vi "Planecontrolscrashworks.vi"() -> ()   [LabVIEW 2015]
uses:
  <vilib>/DAQmx/read.llb/DAQmx Read (Analog Wfm 1Chan NSamp).vi
  <vilib>/DAQmx/create/channels.llb/DAQmx Create Channel (AI-Voltage-Basic).vi
  <vilib>/DAQmx/configure/timing.llb/DAQmx Timing (Sample Clock).vi
  \\hs4.lboro.ac.uk\elhh3/LabVIEW Data/Work/Invictus/Global.vi
  <vilib>/DAQmx/miscellaneous.llb/DAQmx Fill In Error Info.vi
panel:
  in  "stop 4":bool
  out "Crash":bool
  in  "stop 5":bool
  in  "Amplitude":dbl(slide) scale=0.0..5000.0
  in  "stop 3":bool
  in  "stop 2":bool
  in  "stop":bool
  out "Altitude":dbl
  out "Iterations":i32
  out "Light Sensor":dbl
  out "Roll":dbl
  out "Airspeed":dbl
  out "Boolean":bool
  in  "Wing Tips":bool
  out "Previous Speed":dbl
  out "?":bool
  out "?":bool
  out "?":bool
  out "?":bool
  in  "Current Speed":dbl(slide) scale=0.0..400.0
  in  "Roll Slider":dbl(slide) scale=-90.0..90.0
  in  "Fan":bool
  in  "Breaks":bool
  in  "Right Indicator":bool
  in  "Left Indicator":bool
  out "Waveform Graph":waveform(dbl)(graph)
  in  "?":bool
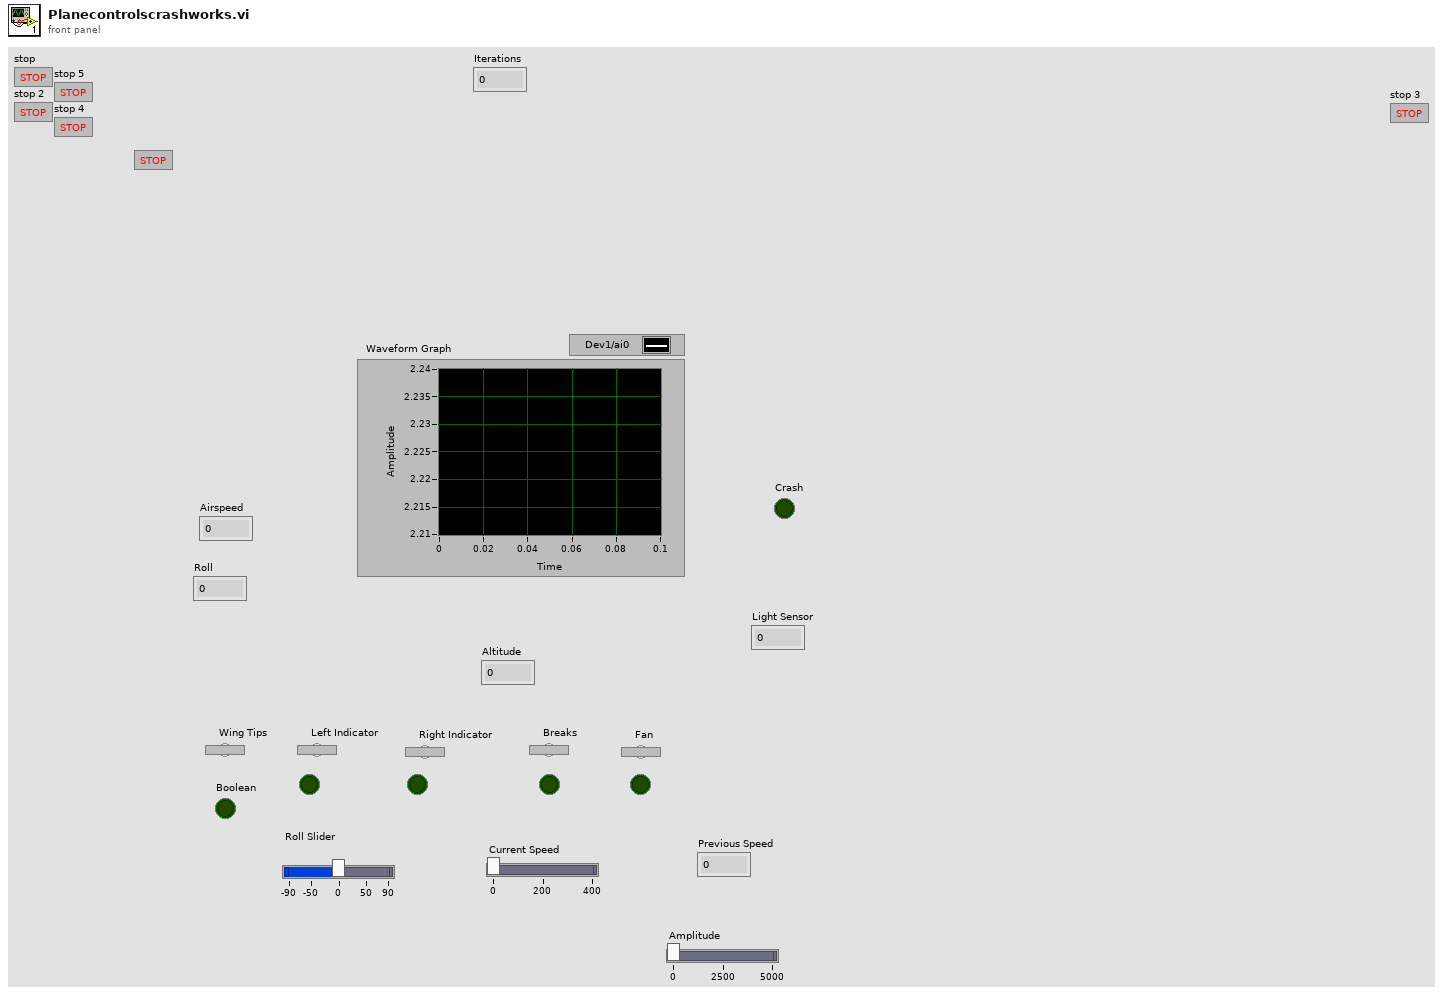
[diagram p1: front panel]
types:
  T1 = cluster{"Airspeed":dbl, "Altitude":dbl, "Vertical Speed":dbl, "Pitch":dbl, "Roll":dbl, "Heading":dbl, "Turn Indicator":dbl, "Latitude":dbl, "Longitude":dbl}
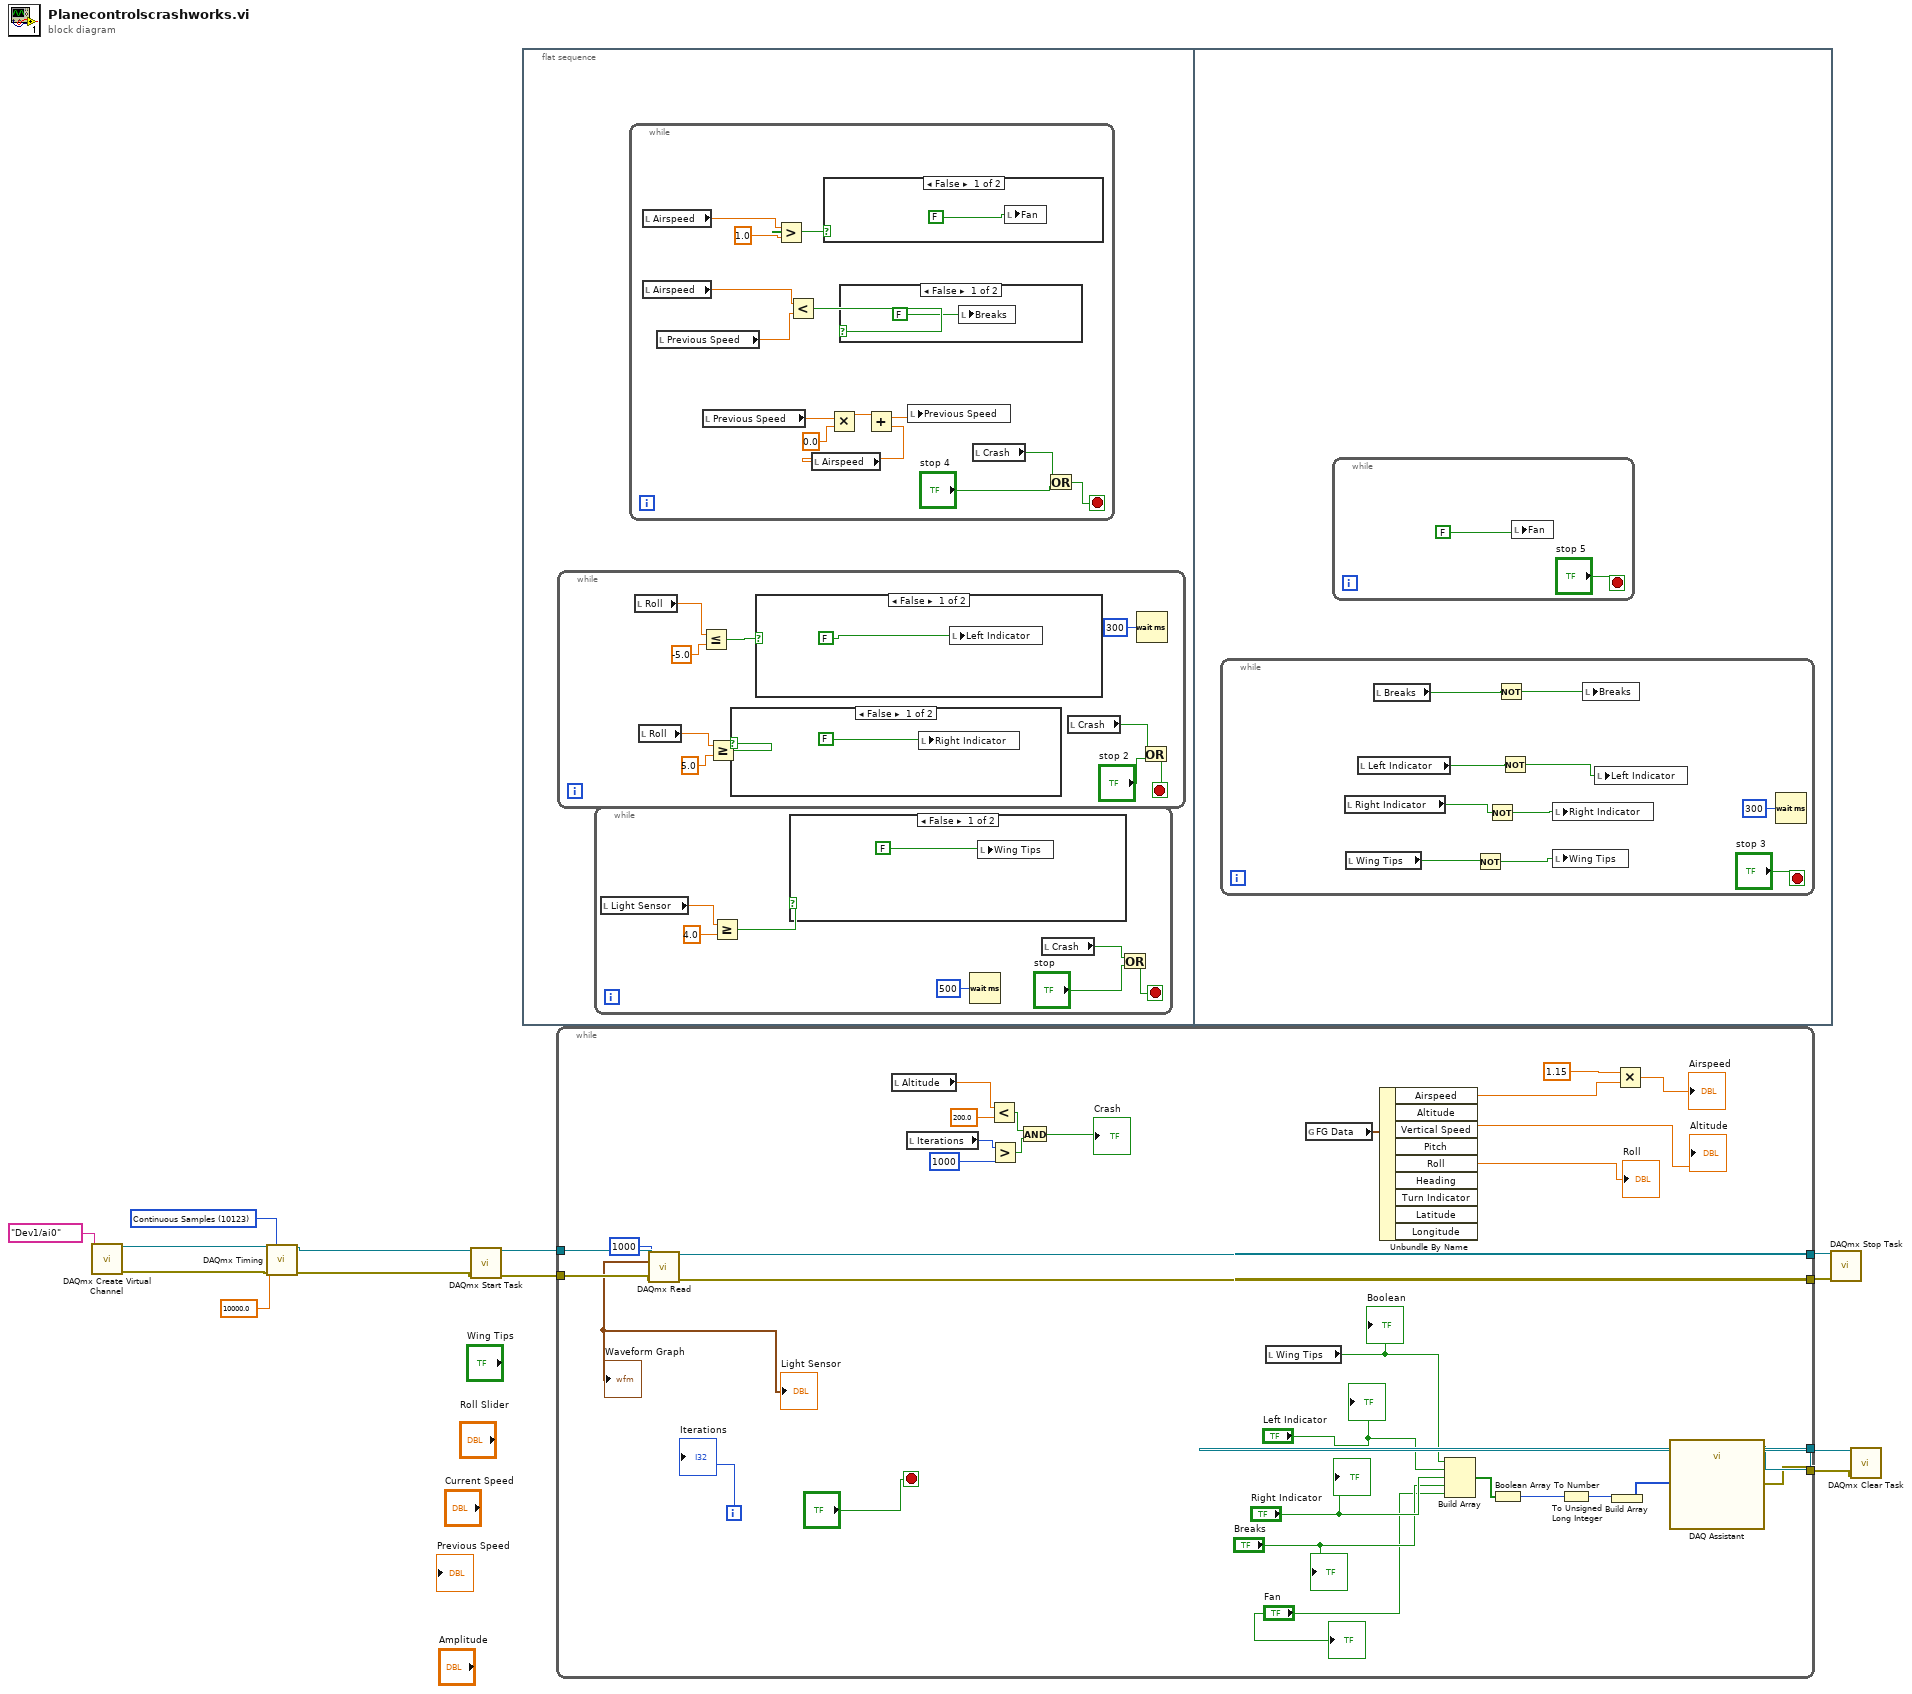
[diagram p0: block diagram]
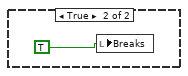
[diagram p2: hidden frame]
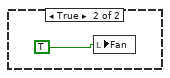
[diagram p3: hidden frame]
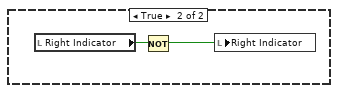
[diagram p4: hidden frame]
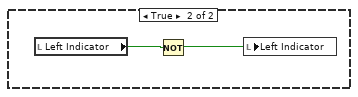
[diagram p5: hidden frame]
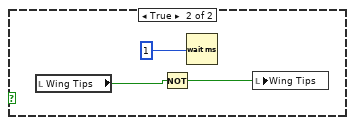
[diagram p6: hidden frame]
diagram:
  w3 = 10123 items=["Finite Samples"=10178, "Continuous Samples"=10123, "Hardware Timed Single Point"=12522] ("sample mode")
  n1 = call-poly <vilib>:"DAQmx Create Virtual Channel.vi"("physical channels"=tag "Dev1/ai0") -> ("task out"=w2:refnum<k21>, "error out"=w5:errorcluster)  [unwired: 13 in]
  n2 = call-poly <vilib>:"DAQmx Timing.vi"("task/channels in"=w2, "sample mode"=w3, "rate"=10000.0, "error in"=w5) -> ("task out"=w9:refnum<k21>, "error out"=w6:errorcluster)  [unwired: 10 in]
  n3 = call <vilib>:"DAQmx Start Task.vi"("task/channels in"=w9, "error in"=w6) -> ("task out"=w8:refnum<k21>, "error out"=w7:errorcluster)  [unwired: 12 in]
  n4 = flat-sequence {
    frame #0 {
      n5 = while {
        stop <- w32 stop-if-true
        n6 = local read "Roll"() -> (w35:dbl)
        n7 = local read "Roll"() -> (w37:dbl)
        n8 = Less Or Equal?(x=w35, y=-5.0) -> (x <= y?=w40:bool)
        n9 = Greater Or Equal?(x=w37, y=5.0) -> (x >= y?=w38:bool)
        n10 = case shown="False" w38 {
          frame False {
            n11 = local write "Right Indicator"(FALSE) -> ()
          }
          frame True {
            n12 = local read "Right Indicator"() -> (w43:bool)
            n13 = Not(x=w43) -> (.not. x?=w44:bool)
            n14 = local write "Right Indicator"(w44) -> ()
          }
        }
        n15 = case shown="False" w40 {
          frame False {
            n16 = local write "Left Indicator"(FALSE) -> ()
          }
          frame True {
            n17 = local read "Left Indicator"() -> (w46:bool)
            n18 = Not(x=w46) -> (.not. x?=w47:bool)
            n19 = local write "Left Indicator"(w47) -> ()
          }
        }
        n20 = local read "Crash"() -> (w34:bool)
        n21 = Wait (ms)(milliseconds to wait=u32 300) -> ()  [unwired: 1 out]
        n22 = Or(x=w34, y="stop 2") -> (x .or. y?=w32:bool)
      }
      n23 = while {
        stop <- w48 stop-if-true
        n24 = local read "Light Sensor"() -> (w52:dbl)
        n25 = Greater Or Equal?(x=w52, y=4.0) -> (x >= y?=w54:bool)
        n26 = case shown="False" w54 {
          frame False {
            n27 = local write "Wing Tips"(FALSE) -> ()
          }
          frame True {
            n28 = local read "Wing Tips"() -> (w57:bool)
            n29 = Not(x=w57) -> (.not. x?=w58:bool)
            n30 = Wait (ms)(milliseconds to wait=u32 1 ("millisecond timer value")) -> ()  [unwired: 1 out]
            n31 = local write "Wing Tips"(w58) -> ()
          }
        }
        n32 = Wait (ms)(milliseconds to wait=u32 500) -> ()  [unwired: 1 out]
        n33 = local read "Crash"() -> (w50:bool)
        n34 = Or(x=w50, y="stop") -> (x .or. y?=w48:bool)
      }
      n35 = while {
        stop <- w14 stop-if-true
        n36 = local read "Airspeed"() -> (w27:dbl)
        n37 = local read "Airspeed"() -> (w23:dbl)
        n38 = local read "Previous Speed"() -> (w17:dbl)
        n39 = local read "Previous Speed"() -> (w21:dbl)
        n40 = Greater?(x=w27, y=1.0 ("x")) -> (0:w26:bool)
        n41 = Less?(x=w23, y=w17) -> (x < y?=w18:bool)
        n42 = local read "Airspeed"() -> (w24:dbl)
        n43 = case shown="False" w26 {
          frame False {
            n44 = local write "Fan"(FALSE) -> ()
          }
          frame True {
            n45 = local write "Fan"(TRUE) -> ()
          }
        }
        n46 = Multiply(x=w21, y=0.0) -> (x*y=w20:dbl)
        n47 = case shown="False" w18 {
          frame False {
            n48 = local write "Breaks"(FALSE) -> ()
          }
          frame True {
            n49 = local write "Breaks"(TRUE) -> ()
          }
        }
        n50 = Add(x=w20, y=w24) -> (x+y=w19:dbl)
        n51 = local write "Previous Speed"(w19) -> ()
        n52 = local read "Crash"() -> (w16:bool)
        n53 = Or(x=w16, y="stop 4") -> (x .or. y?=w14:bool)
      }
    }
    frame #1 {
      n54 = while {
        stop <- "stop 3" stop-if-true
        n55 = local read "Right Indicator"() -> (w64:bool)
        n56 = local read "Wing Tips"() -> (w62:bool)
        n57 = local read "Left Indicator"() -> (w66:bool)
        n58 = local read "Breaks"() -> (w68:bool)
        n59 = Not(x=w62) -> (.not. x?=w61:bool)
        n60 = Not(x=w64) -> (.not. x?=w63:bool)
        n61 = Not(x=w68) -> (.not. x?=w67:bool)
        n62 = Not(x=w66) -> (.not. x?=w65:bool)
        n63 = local write "Right Indicator"(w63) -> ()
        n64 = local write "Wing Tips"(w61) -> ()
        n65 = local write "Breaks"(w67) -> ()
        n66 = local write "Left Indicator"(w65) -> ()
        n67 = Wait (ms)(milliseconds to wait=u32 300) -> ()  [unwired: 1 out]
      }
      n68 = while {
        stop <- "stop 5" stop-if-true
        n69 = local write "Fan"(FALSE) -> ()
      }
    }
  }
  n70 = while {
    tunnel: w7 -> [w102]
    tunnel: w8 -> [w101]
    tunnel: [w100] -> w10
    tunnel: [w99] -> w11
    tunnel: [w96] -> w12
    tunnel: [w95] -> w13
    i -> [w80]
    stop <- "?" stop-if-true
    n71 = call-poly <vilib>:"DAQmx Read.vi"("task/channels in"=w101, "number of samples per channel"=1000, "error in"=w102) -> ("task out"=w99:refnum<k21>, "data"=→"Waveform Graph" →"Light Sensor":waveform(dbl), "error out"=w100:errorcluster)  [unwired: 10 in]
    n72 = local read "Altitude"() -> (w71:dbl)
    n73 = local read "Iterations"() -> (w78:i32)
    n74 = Less?(x=w71, y=200.0) -> (x < y?=w74:bool)
    n75 = Greater?(x=w78, y=1000) -> (0:w75:bool)
    n76 = And(x=w74, y=w75) -> (x .and. y?=→"Crash":bool)
    n77 = local read "Wing Tips"() -> (w87:bool)
    "Boolean" <- w87
    n78 = global read "Global.vi" "FG Data"() -> (w86:T1)
    n79 = Unbundle By Name(w86) -> ("Airspeed"=w84:dbl, "Altitude"=→"Altitude":dbl, "Roll"=→"Roll":dbl)  [unwired: 6 out]
    n80 = Build Array(w87, "Left Indicator", "Right Indicator", "Breaks", "Fan") -> (w94:bool[])
    n81 = Boolean Array To Number(Boolean array=w94) -> (number=w97:u32)
    n82 = To Unsigned Long Integer(number=w97) -> (unsigned 32bit integer=w93:u32)
    n83 = Build Array(w93) -> (w92:u32[])
    n84 = Multiply(x=1.15, y=w84) -> (x*y=→"Airspeed":dbl)
    n85 = call "DAQ Assistant"("data"=w92) -> ("task out"=w96:refnum<k21>, "error out"=w95:errorcluster)  [unwired: 17 in]
    "?" <- "Left Indicator"
    "?" <- "Right Indicator"
    "?" <- "Breaks"
    "?" <- "Fan"
    "Iterations" <- w80
  }
  n86 = call <vilib>:"DAQmx Stop Task.vi"("task/channels in"=w11, "error in"=w10) -> ()  [unwired: 12 in, 2 out]
  n87 = call <vilib>:"DAQmx Clear Task.vi"("task in"=w12, "error in"=w13) -> ()  [unwired: 13 in, 1 out]
